vi "Robot Global Data.vi"() -> ()   [LabVIEW 2011]
doc: "This global VI can contain as many global variables as you need. Place a control on the panel, give it a good name. To read or write to it from a VI, drag the icon to the diagram of that VI. You can also drag from the project. Click on the node to change which global you access. You shouldn't have multiple locations writing to a global or it will cause a race-condition."
uses:
  <vilib>/Rock Robotics/WPI/DriverStation/WPI_DriverStationRobotMode.ctl
  TypeDefs/Dashboard Data TypeDef.ctl
panel:
  in  "Drive Around Mode?":bool
  in  "Coop Bridge":dbl=2600.0
  in  "Light On?":bool
  in  "Arm Down?":bool
  in  "Number of Balls":i32
  in  "De-Jam?":bool
  in  "Shooting Manual Override?":bool
  in  "FIRE!!!!!!":bool
  in  "Auton Elapsed Time":dbl
  in  "Top Hoop Back of Key":dbl=2100.0
  in  "Top Hoop Front of Key":dbl=1900.0
  in  "Top Hoop Other Side of Barrier":dbl=2700.0
  in  "StLouis Dashboard Data":T1={"Number of Balls"=0, "Shooting Manual Override?"=FALSE, "Bridge Mode?"=FALSE, "Shooter"=TRUE, "Shooter At Speed?"=TRUE, "Aligning Mode?"=FALSE}
  in  "Real Hoop Free Throw":dbl=2200.0
  in  "Real Hoop 3 Pointer":dbl=2600.0
  in  "Top Hoop Key Speed":dbl=2000.0
  in  "Fender Speed":dbl=1300.0
  out "Shooter at Speed?":bool=TRUE
  out "Autonomous":T2={"Autonomous Delay"=0.0, "Autonomous Mode"=enum."Middle of Key (SEA)"}
  out "Ball Count":T3
  in  "Robot Mode":T4=enum."Finish"
  in  "Set RPM":dbl
  out "Current RPM":dbl
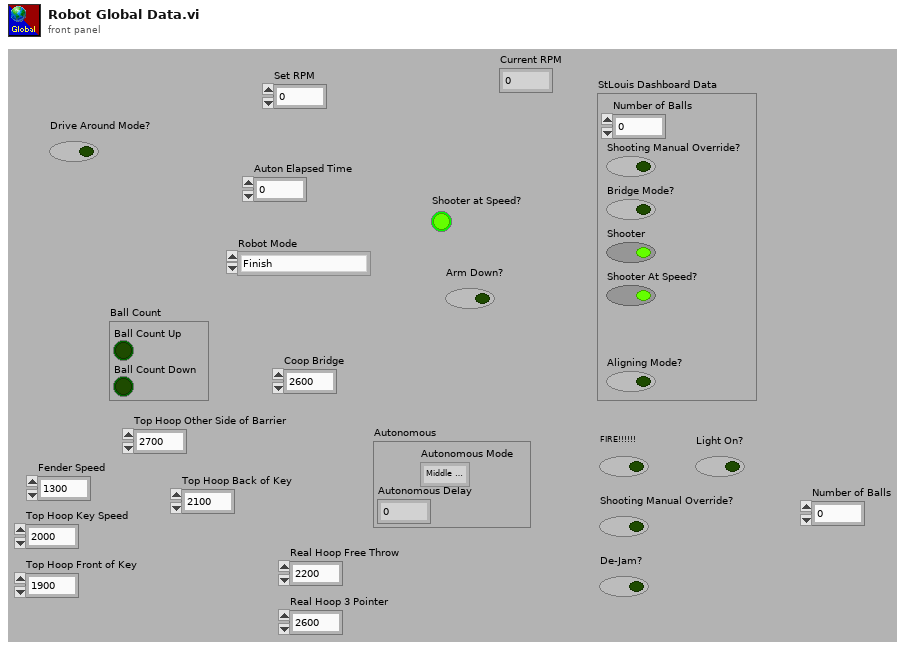
[diagram p1: front panel]
types:
  T1 = typedef "Dashboard Data TypeDef.ctl" = cluster{"Number of Balls":i32, "Shooting Manual Override?":bool, "Bridge Mode?":bool, "Shooter":bool, "Shooter At Speed?":bool, "Aligning Mode?":bool}
  T2 = cluster{"Autonomous Delay":dbl, "Autonomous Mode":enum16{"Front Of Key", "Middle of Key (SEA)", "Back of Key", "Bridge", "Disable"}}
  T3 = cluster{"Ball Count Up":bool, "Ball Count Down":bool}
  T4 = typedef "WPI_DriverStationRobotMode.ctl" = enum16{"Autonomous Disabled", "Autonomous Enabled", "Teleop Disabled", "Teleop Enabled", "Timeout", "Finish"}
diagram:
